vi "Current Write Array.vi"(8 "error in":errorcluster, 10 "Current AV":dbl[](array[numeric]), 11 "Cycler in":refnum<class "Cycler.lvclass">) -> (0 "error out":errorcluster, 3 "Cycler out":refnum<class "Cycler.lvclass">)   [LabVIEW 2023, in "Cycler.lvclass"]
uses:
  Cycler.lvclass
  Cycler.lvclass/Cycler.ctl
  Low Level Capabilities/Current/Current Actual Value/Current Actual Value.lvclass
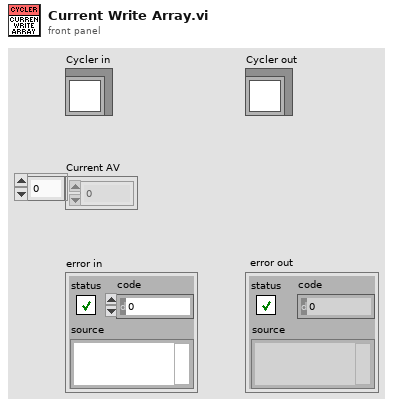
[diagram p1: front panel]
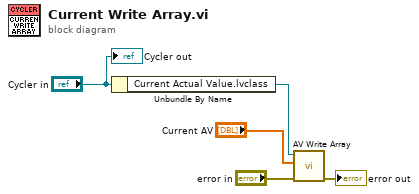
[diagram p0: block diagram]
diagram:
  n1 = Unbundle By Name("Cycler in") -> ("Current Actual Value.lvclass"=w5:refnum<class "Current Actual Value.lvclass">)
  n2 = call-dynamic "AV Write Array.vi"("error in"="error in", "Current AV"="Current AV", "Current Actual Value in"=w5) -> ("error out"=→"error out":errorcluster)  [unwired: 7 in, 1 out]
  "Cycler out" <- "Cycler in"
